vi "TestPath.vi"(8 "error in (no error)":errorcluster, 11 "Example Instrument in":refnum<class "Example Instrument.lvclass">) -> (0 "error out":errorcluster, 3 "Example Instrument out":refnum<class "Example Instrument.lvclass">)   [LabVIEW 2016, in "Example Instrument.lvclass"]
uses:
  Example Instrument.lvclass
  <userlib>/LevyLab/Levylab Instruments/SMOs/Instrument/Typedefs/Configuration--Cluster.ctl
  <userlib>/LevyLab/Levylab Instruments/SMOs/Instrument/Typedefs/HW Configuration--Cluster.ctl
  <userlib>/LevyLab/Levylab Instruments/SMOs/Instrument/Typedefs/SMO Configuration--Cluster.ctl
  <userlib>/LevyLab/Levylab Instruments/SMOs/Instrument/Typedefs/SMO RC Type--enum.ctl
  <userlib>/LevyLab/Levylab Instruments/SMOs/Instrument/Typedefs/DSC Configuration--Cluster.ctl
  <userlib>/LevyLab/Levylab Instruments/SMOs/Configuration/Configuration.lvclass
  <userlib>/LevyLab/Levylab Instruments/SMOs/Instrument/Instrument.lvclass
panel:
  in  "Configuration":T1={"Hardware"={"Address"="", "Type"="", "COM Type"=""}, "SMO"={"Address"="", "Port"=0, "RC Type"=enum."RC"}, "DSC"={"Process Name"="instrument"}}
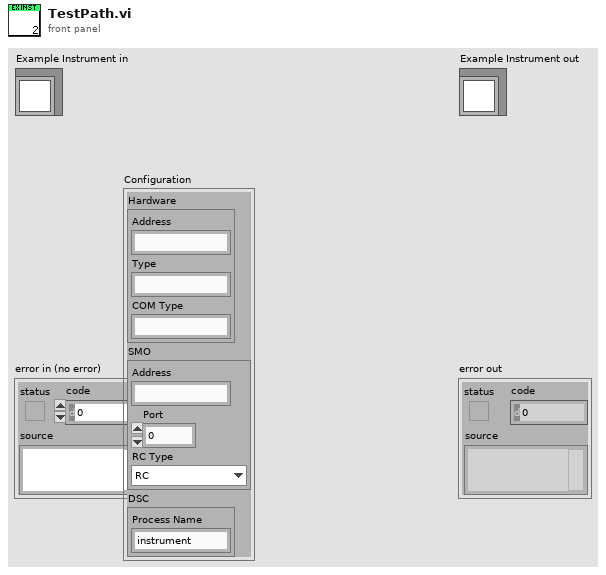
[diagram p1: front panel]
types:
  T1 = typedef "Instrument.lvclass/Configuration--Cluster.ctl" = cluster{"Hardware":T2, "SMO":T3, "DSC":T5}
  T2 = typedef "Instrument.lvclass/HW Configuration--Cluster.ctl" = cluster{"Address":string, "Type":string, "COM Type":string}
  T3 = typedef "Instrument.lvclass/SMO Configuration--Cluster.ctl" = cluster{"Address":string, "Port":u16, "RC Type":T4}
  T4 = typedef "Instrument.lvclass/SMO RC Type--enum.ctl" = enum16{"RC", "STM", "ZMQ"}
  T5 = typedef "Instrument.lvclass/DSC Configuration--Cluster.ctl" = cluster{"Process Name":string}
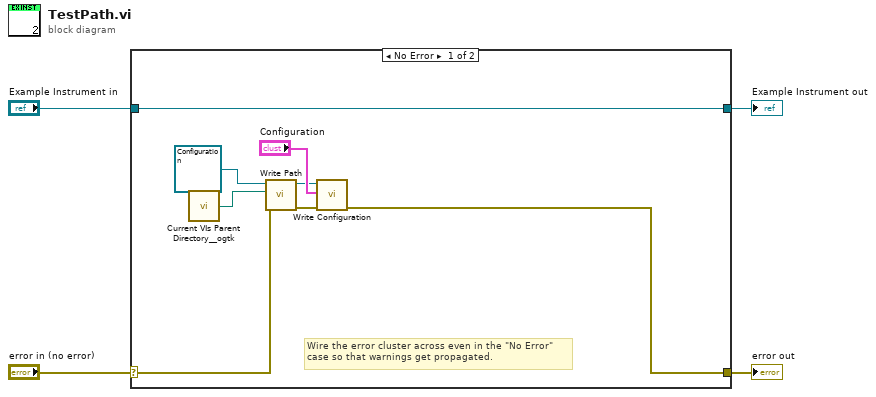
[diagram p0: block diagram]
diagram:
  n1 = case shown="No Error" "error in (no error)" {
    selector: "error in (no error)" -> [w6 w14]
    tunnel: [w5 w14] -> w3
    tunnel: [w12 w13] -> w1
    tunnel: "Example Instrument in" -> [w12 w13]
    frame No Error {
      # "Wire the error cluster across even in the \"No Error\"\ncase so that warnings get propagated."
      n2 = call <userlib>:"Current VIs Parent Directory__ogtk.vi"() -> ("Parent Directory (+ Relative)"=w11:path)  [unwired: 5 in]
      n3 = call-dynamic "Write Path.vi"("error in (no error)"=w6, "Path"=w11, "Configuration in"=refnum<class "Configuration.lvclass"> refnum) -> ("error out"=w8:errorcluster, "Configuration out"=w9:refnum<class "Configuration.lvclass">)  [unwired: 7 in]
      n4 = call <userlib>:"Write Configuration.vi"("error in (no error)"=w8, "Variant"="Configuration", "Configuration in"=w9) -> ("error out"=w5:errorcluster)  [unwired: 7 in, 1 out]
    }
    frame Error {
    }
  }
  "error out" <- w3
  "Example Instrument out" <- w1
